vi "MasterSlaveDAQ.vi"() -> ()   [LabVIEW 2014]
doc: "Use this template to build a user interface event handler design pattern. Use this pattern for dialog boxes and other user interfaces. You also can create and execute user-defined events that the VI can handle the same way as user interface events."
uses:
  subVIs/MasterState.ctl
  subVIs/SlaveStateData.ctl
  subVIs/SlaveState.ctl
  <vilib>/Utility/error.llb/DialogType.ctl
  <vilib>/DAQmx/create/channels.llb/DAQmx Create Channel (AI-Voltage-Basic).vi
  <vilib>/DAQmx/configure/timing.llb/DAQmx Timing (Sample Clock).vi
  <vilib>/DAQmx/read.llb/DAQmx Read (Analog Wfm 1Chan NSamp).vi
  <resource>/objmgr/daqmx.rc
panel:
  in  "File Path":path
  in  "Acquire Data":bool
  in  "Log Data":bool
  in  "File Comment":string
  in  "DAQ Parameters":T1={"physical channels"="", "maximum value"=5.0, "minimum value"=-5.0, "rate"=1000.0, "read period"=0.5} {"read period" format="%0.2f"; "rate" format="%0.2f"; "minimum value" format="%0.2f"; "maximum value" format="%0.2f"}
  out "Waveform Chart":waveform(dbl)(graph)
  in  "quit":bool
  # "V"
  # "V"
  # "Hz"
  # "s"
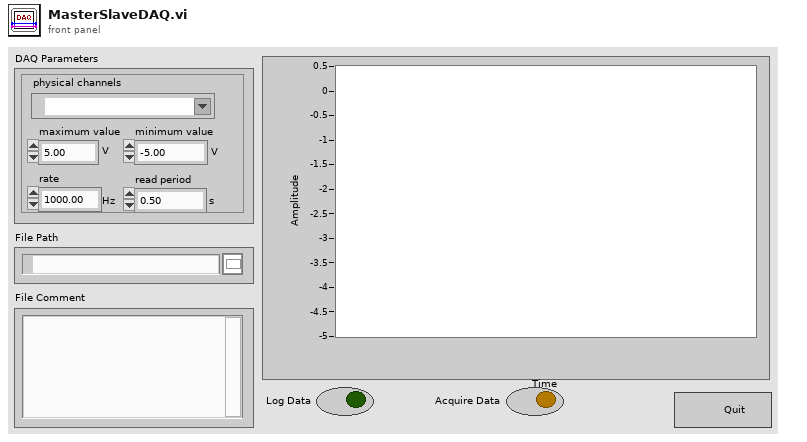
[diagram p1: front panel]
types:
  T1 = cluster{"physical channels":tag, "maximum value":dbl, "minimum value":dbl, "rate":dbl, "read period":dbl}
  T2 = typedef "SlaveState.ctl" = enum16{"Init", "Idle", "CheckError", "Finalize", "StartDAQ", "AcquireAndLog", "StopDAQ", "UpdateFile"}
  T3 = typedef "SlaveStateData.ctl" = cluster{"New State":T2, "DAQ Ref":refnum<k21>, "File Ref":refnum<file>}
  T4 = typedef "MasterState.ctl" = enum16{"Init", "Idle", "CheckError", "Finalize", "ConfigDAQ", "StartDAQ", "AcquireAndLog", "StopDAQ", "ClearDAQ", "OpenFile", "CloseFile"}
  T5 = typedef "DialogType.ctl" = u16
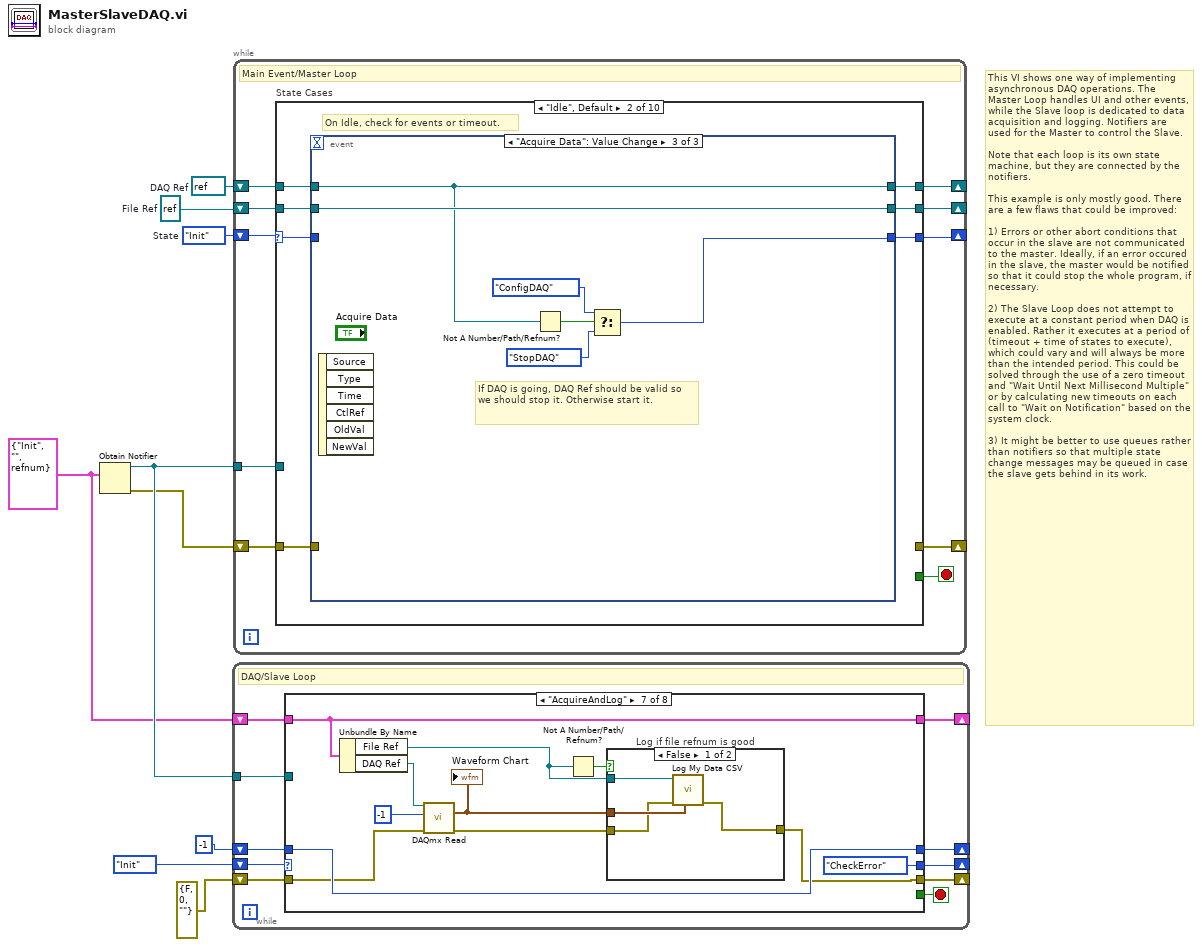
[diagram p0: block diagram]
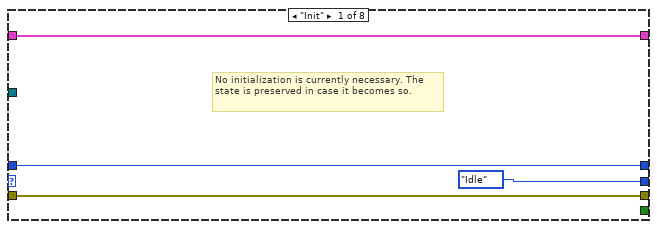
[diagram p2: hidden frame]
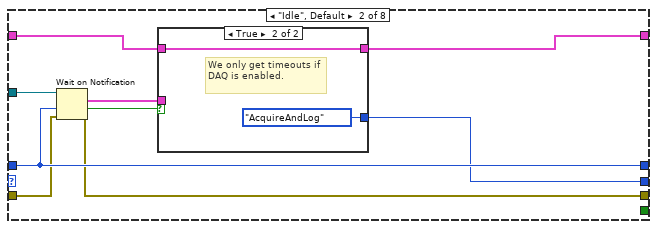
[diagram p3: hidden frame]
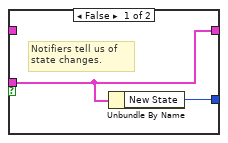
[diagram p4: hidden frame]
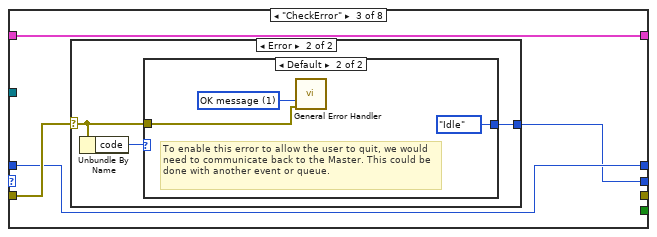
[diagram p5: hidden frame]
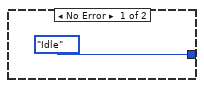
[diagram p6: hidden frame]
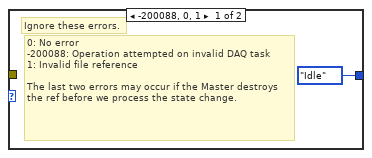
[diagram p7: hidden frame]
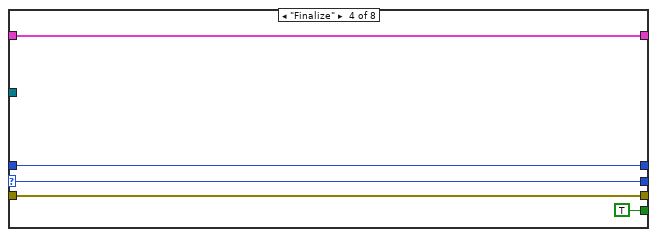
[diagram p8: hidden frame]
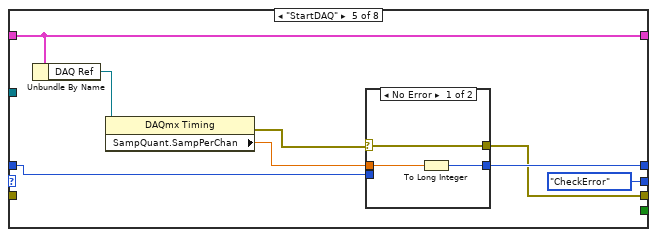
[diagram p9: hidden frame]
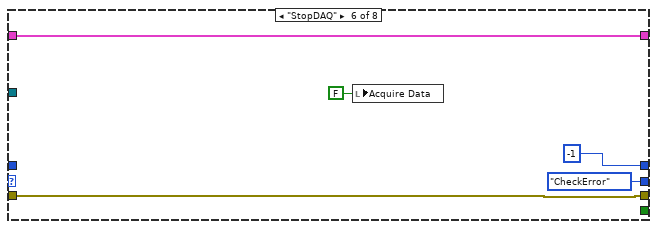
[diagram p11: hidden frame]
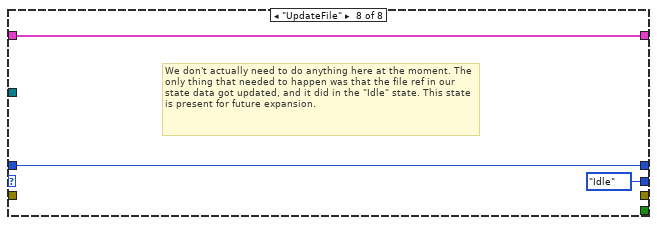
[diagram p13: hidden frame]
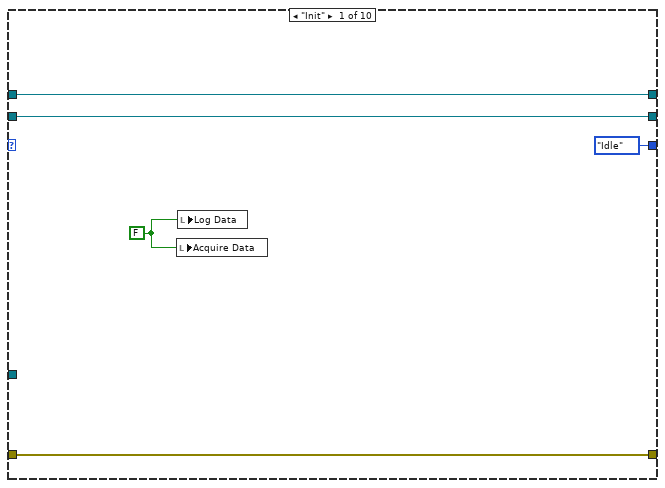
[diagram p14: hidden frame]
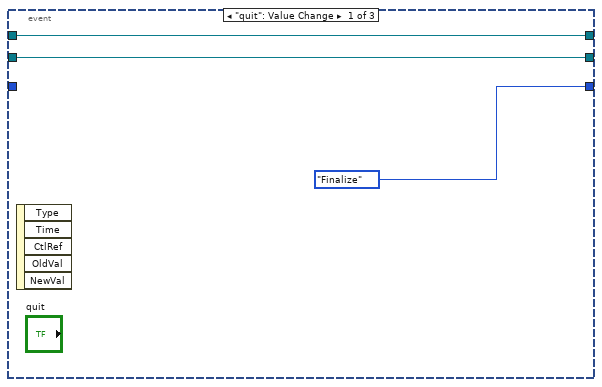
[diagram p15: hidden frame]
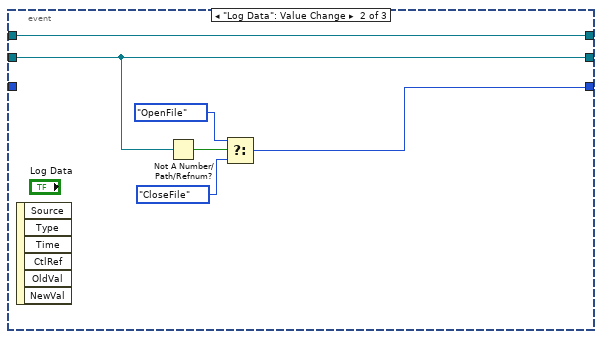
[diagram p16: hidden frame]
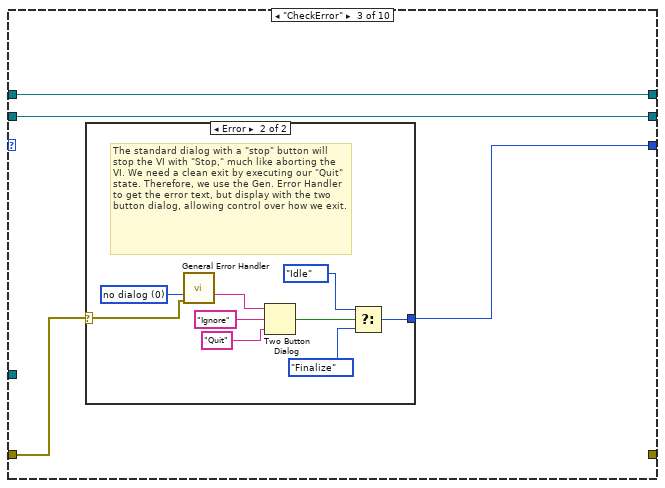
[diagram p17: hidden frame]
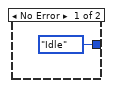
[diagram p18: hidden frame]
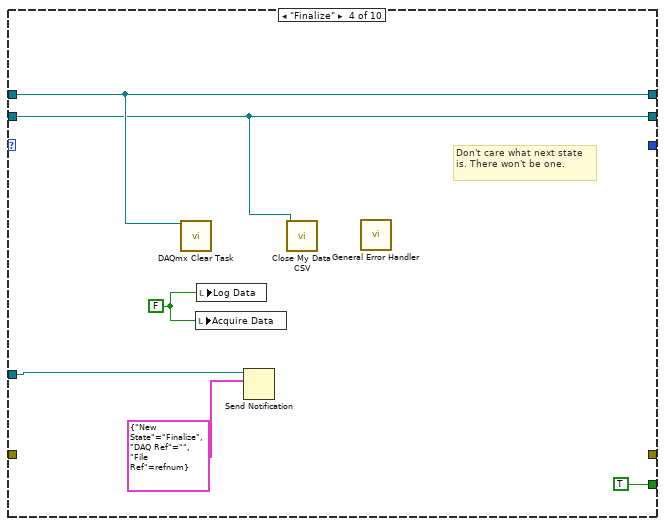
[diagram p19: hidden frame]
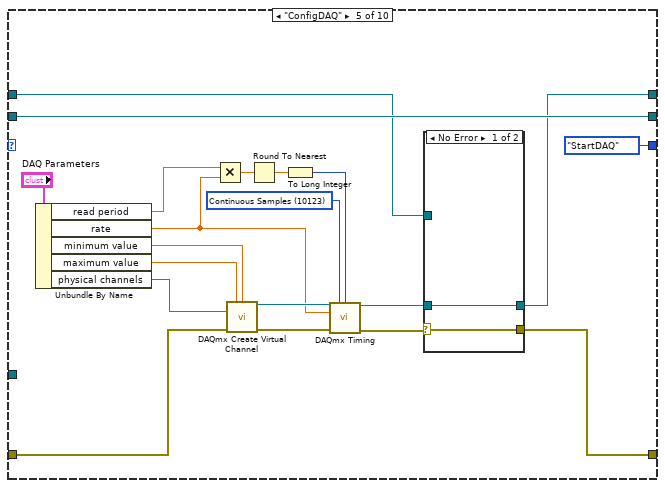
[diagram p20: hidden frame]
diagram:
  w4 = T3 {"New State"=enum."Init", "DAQ Ref"="", "File Ref"=refnum}
  w7 = refnum<file> refnum  # File Ref
  w8 = refnum<k21> refnum  # DAQ Ref
  w9 = MasterState."Init"  # State
  # "This VI shows one way of implementing asynchronous DAQ operations. The Master Loop handles UI and other events, while the Slave loop is dedicated to data acquisition and logging. Notifiers are used for the Master to control the Slave.\n\nNote that each loop is its own state machine, but they are connected by the notifiers.\n\nThis example is only mostly good. There are a few flaws that could be improved:\n\n1) Errors or other abort conditions that occur in the slave are not communicated to the master. Ideally, if an error occured in the slave, the master would be notified so that it could stop the whole program, if necessary.\n\n2) The Slave Loop does not attempt to execute at a constant period when DAQ is enabled. Rather it executes at a period of (timeout + time of states to execute), which could vary and will always be more than the intended period. This could be solved through the use of a zero timeout and \"Wait Until Next Millisecond Multiple\" or by calculating new timeouts on each call to \"Wait on Notification\" based on the system clock.\n\n3) It might be better to use queues rather than notifiers so that multiple state change messages may be queued in case the slave gets behind in its work."
  n1 = Obtain Notifier(notification data type=w4) -> (notifier out=w6:refnum<notifier>, error out=w2:errorcluster)  [unwired: 3 in, 1 out]
  n2 = while {
    tunnel: w6 -> [w18]
    shift-right: [w17] -> _
    shift-left: SlaveState."Init" ("State") -> [w19]
    shift-right: [w13] -> _
    shift-left: w4 -> [w16]
    shift-right: [w14] -> _
    shift-left: -1 -> [w15]
    shift-right: [w11] -> _
    shift-left: errorcluster {"status"=FALSE, "code"=0, "source"=""} ("error out") -> [w12]
    stop <- w10 stop-if-true
    # "DAQ/Slave Loop"
    n3 = case shown="\"AcquireAndLog\"" w19 {
      selector: w19 -> [_ _ _ w50 _ _ _ _]
      tunnel: w18 -> [_ w32 _ _ _ _ _ _]
      tunnel: [SlaveState."Idle" ("New State") w25 w37 w50 SlaveState."CheckError" ("State") SlaveState."CheckError" ("State") SlaveState."CheckError" ("State") SlaveState."Idle" ("State")] -> w17
      tunnel: w16 -> [w21 w27 w40 w52 w57 w71 w76 w90]
      tunnel: w15 -> [w22 w31 w38 w51 w59 _ w77 w89]
      tunnel: [w22 w31 w38 w51 w60 -1 w77 w89] -> w14
      tunnel: [w21 w24 w40 w52 w57 w71 w76 w90] -> w13
      tunnel: w12 -> [w20 w29 w39 w49 _ w67 w74 _]
      tunnel: [w20 w30 _ w49 w58 w67 w73 _] -> w11
      tunnel: [_ _ _ TRUE _ _ _ _] -> w10
      frame "Init" {
        # "No initialization is currently necessary. The state is preserved in case it becomes so."
      }
      frame "Idle", Default {
        n4 = Wait on Notification(notifier=w32, timeout in ms (-1)=w31, error in (no error)=w29) -> (notification=w26:T3, timed out?=w28:bool, error out=w30:errorcluster)  [unwired: 1 in, 1 out]
        n5 = case shown="True" w28 {
          tunnel: w27 -> [_ w36]
          tunnel: w26 -> [w33 _]
          tunnel: [w34 SlaveState."AcquireAndLog" ("New State")] -> w25
          tunnel: [w33 w36] -> w24
          frame False {
            # "Notifiers tell us of state changes."
            n6 = Unbundle By Name(w33) -> ("New State"=w34:T2)
          }
          frame True {
            # "We only get timeouts if DAQ is enabled."
          }
        }
      }
      frame "CheckError" {
        n7 = case shown="Error" w39 {
          selector: w39 -> [_ w43]
          tunnel: [SlaveState."Idle" ("State") w44] -> w37
          frame No Error {
          }
          frame Error {
            n8 = Unbundle By Name(w43) -> ("code"=w42:i32)
            n9 = case shown="Default" w42 {
              tunnel: [SlaveState."Idle" ("State") SlaveState."Idle" ("State")] -> w44
              tunnel: w43 -> [_ w47]
              frame -200088, 0, 1 {
                # "0: No error\n-200088: Operation attempted on invalid DAQ task\n1: Invalid file reference\n\nThe last two errors may occur if the Master destroys the ref before we process the state change."
                # "Ignore these errors."
              }
              frame Default {
                w48 = T5 1 items=["no dialog", "OK message", "continue or stop message", "OK message + warnings", "continue/stop + warnings"] ("type of dialog (OK msg:1)")
                # "To enable this error to allow the user to quit, we would need to communicate back to the Master. This could be done with another event or queue."
                n10 = call <vilib>:"General Error Handler.vi"("type of dialog (OK msg:1)"=w48, "error in (no error)"=w47) -> ()  [unwired: 9 in, 5 out]
              }
            }
          }
        }
      }
      frame "Finalize" {
      }
      frame "StartDAQ" {
        n11 = Unbundle By Name(w57) -> ("DAQ Ref"=w56:refnum<k21>)
        n12 = property class="DAQmx Timing"(reference=w56) -> (error out=w54:errorcluster, "SampQuant.SampPerChan"=w61:dbl)  [unwired: 1 in, 1 out]
        n13 = case shown="No Error" w54 {
          selector: w54 -> [w62 w66]
          tunnel: w61 -> [w64 _]
          tunnel: [w63 w65] -> w60
          tunnel: [w62 w66] -> w58
          tunnel: w59 -> [_ w65]
          frame No Error {
            n14 = To Long Integer(number=w64) -> (32bit integer=w63:i32)
          }
          frame Error {
          }
        }
      }
      frame "StopDAQ" {
        n15 = local write "Acquire Data"(FALSE ("Acquire Data")) -> ()
      }
      frame "AcquireAndLog" {
        n16 = Unbundle By Name(w76) -> ("File Ref"=w72:refnum<file>, "DAQ Ref"=w75:refnum<k21>)
        n17 = call-poly <vilib>:"DAQmx Read.vi"("task/channels in"=w75, "number of samples per channel"=-1, "error in"=w74) -> ("data"=w78:waveform(dbl), "error out"=w79:errorcluster)  [unwired: 10 in, 1 out]
        "Waveform Chart" <- w78
        n18 = Not A Number/Path/Refnum?(number/path/refnum=w72) -> (NaN/Path/Refnum?=w80:bool)
        n19 = case "Log if file refnum is good" shown="False" w80 {
          tunnel: w79 -> [w83 w87]
          tunnel: w72 -> [w86 _]
          tunnel: w78 -> [w85 _]
          tunnel: [w84 w87] -> w73
          frame False {
            n20 = call "Log My Data CSV.vi"("Data"=w85, "error in"=w83, "file refnum"=w86) -> ("error out"=w84:errorcluster)  [unwired: 7 in, 1 out]
          }
          frame True {
          }
        }
      }
      frame "UpdateFile" {
        # "We don't actually need to do anything here at the moment. The only thing that needed to happen was that the file ref in our state data got updated, and it did in the \"Idle\" state. This state is present for future expansion."
      }
    }
  }
  n21 = while {
    shift-right: [w99] -> _
    shift-left: w9 -> [w100]
    shift-right: [w98] -> _
    shift-left: w8 -> [w97]
    shift-right: [w96] -> _
    shift-left: w7 -> [w95]
    shift-right: [w94] -> _
    shift-left: w2 -> [w93]
    tunnel: w6 -> [w91]
    stop <- w92 stop-if-true
    # "Main Event/Master Loop"
    n22 = case "State Cases" shown="\"Idle\", Default" w100 {
      selector: w100 -> [_ w112 _ _ _ _ _ _ _ _]
      tunnel: [MasterState."Idle" ("State") w111 w129 _ MasterState."StartDAQ" ("State") MasterState."CheckError" ("State") MasterState."ClearDAQ" ("State") MasterState."CheckError" ("State") MasterState."CheckError" ("State") MasterState."CheckError" ("State")] -> w99
      tunnel: [w105 w108 w131 w146 w158 w174 w188 refnum<k21> refnum ("DAQ Ref") w204 w230] -> w98
      tunnel: w97 -> [w105 w107 w131 w146 w159 w174 w188 w198 w204 w230]
      tunnel: [w104 w110 w130 w145 w167 w177 w195 w200 w215 w234] -> w96
      tunnel: w95 -> [w104 w109 w130 w145 w167 w177 w195 w200 w205 w237]
      tunnel: [w101 _ _ _ w156 w178 w190 w196 w214 w227] -> w94
      tunnel: w93 -> [w101 w106 w128 _ w148 w175 w187 w197 w211 w233]
      tunnel: [_ _ _ TRUE _ _ _ _ _ _] -> w92
      tunnel: w91 -> [_ _ _ w143 _ w182 w194 _ w208 w226]
      frame "Init" {
        w102 = FALSE
        n23 = local write "Acquire Data"(w102) -> ()
        n24 = local write "Log Data"(w102) -> ()
      }
      frame "Idle", Default {
        # "On Idle, check for events or timeout."
        # "States"
        n25 = event shown="[2] \"Acquire Data\": Value Change" {
          selector: _ -> [_ _ _]
          dyn-events: _ -> [_ _ _]
          timeout: _ -> [_ _ _]
          tunnel: w112 -> [_ _ _]
          tunnel: [MasterState."Finalize" ("State") w116 w122] -> w111
          tunnel: [w114 w119 w127] -> w110
          tunnel: w109 -> [w114 w119 w127]
          tunnel: [w115 w121 w125] -> w108
          tunnel: w107 -> [w115 w121 w125]
          tunnel: w106 -> [_ _ _]
          event "quit": Value Change {
            n26 = event-data() -> ()  [unwired: 1 in, 5 out]
          }
          event "Log Data": Value Change {
            n27 = event-data() -> ()  [unwired: 1 in, 6 out]
            n28 = Not A Number/Path/Refnum?(number/path/refnum=w119) -> (NaN/Path/Refnum?=w120:bool)
            n29 = Select(t=MasterState."OpenFile" ("State"), s=w120, f=MasterState."CloseFile" ("State")) -> (s? t:f=w116:T4)
          }
          event "Acquire Data": Value Change {
            # "If DAQ is going, DAQ Ref should be valid so we should stop it. Otherwise start it."
            n30 = event-data() -> ()  [unwired: 1 in, 6 out]
            n31 = Not A Number/Path/Refnum?(number/path/refnum=w125) -> (NaN/Path/Refnum?=w126:bool)
            n32 = Select(t=MasterState."ConfigDAQ" ("State"), s=w126, f=MasterState."StopDAQ" ("State")) -> (s? t:f=w122:T4)
          }
        }
      }
      frame "CheckError" {
        n33 = case shown="Error" w128 {
          selector: w128 -> [_ w133]
          tunnel: [MasterState."Idle" ("State") w134] -> w129
          frame No Error {
          }
          frame Error {
            w141 = T5 0 items=["no dialog", "OK message", "continue or stop message", "OK message + warnings", "continue/stop + warnings"] ("type of dialog (OK msg:1)")
            # "The standard dialog with a \"stop\" button will stop the VI with \"Stop,\" much like aborting the VI. We need a clean exit by executing our \"Quit\" state. Therefore, we use the Gen. Error Handler to get the error text, but display with the two button dialog, allowing control over how we exit."
            n34 = call <vilib>:"General Error Handler.vi"("type of dialog (OK msg:1)"=w141, "error in (no error)"=w133) -> ("message"=w140:string)  [unwired: 9 in, 4 out]
            n35 = Two Button Dialog(message=w140, 1:"Quit" ("F button name (\"Cancel\")"), 2:"Ignore" ("T button name (\"OK\")")) -> (T button?=w137:bool)
            n36 = Select(t=MasterState."Idle" ("State"), s=w137, f=MasterState."Finalize" ("State")) -> (s? t:f=w134:T4)
          }
        }
      }
      frame "Finalize" {
        w144 = FALSE
        # "Don't care what next state is. There won't be one."
        n37 = call <vilib>:"DAQmx Clear Task.vi"("task in"=w146) -> ()  [unwired: 14 in, 1 out]
        n38 = local write "Acquire Data"(w144) -> ()
        n39 = local write "Log Data"(w144) -> ()
        n40 = Send Notification(notification=T3 {"New State"=enum."Finalize", "DAQ Ref"="", "File Ref"=refnum}, notifier=w143) -> ()  [unwired: 1 in, 2 out]
        n41 = call "Close My Data CSV.vi"("file refnum"=w145) -> ()  [unwired: 10 in, 1 out]
        n42 = call <vilib>:"General Error Handler.vi"() -> ()  [unwired: 11 in, 5 out]
      }
      frame "ConfigDAQ" {
        w164 = 10123 items=["Finite Samples"=10178, "Continuous Samples"=10123, "Hardware Timed Single Point"=12522] ("sample mode")
        n43 = Unbundle By Name("DAQ Parameters") -> ("read period"=w153:dbl, "rate"=w152:dbl, "minimum value"=w151:dbl, "maximum value"=w150:dbl, "physical channels"=w149:tag)
        n44 = Multiply(x=w153, y=w152) -> (x*y=w163:dbl)
        n45 = call-poly <vilib>:"DAQmx Create Virtual Channel.vi"("maximum value"=w150, "minimum value"=w151, "physical channels"=w149, "error in"=w148) -> ("task out"=w166:refnum<k21>, "error out"=w165:errorcluster)  [unwired: 10 in]
        n46 = Round To Nearest(number=w163) -> (nearest integer value=w162:dbl)
        n47 = To Long Integer(number=w162) -> (32bit integer=w161:i32)
        n48 = call-poly <vilib>:"DAQmx Timing.vi"("task/channels in"=w166, "sample mode"=w164, "samples per channel"=w161, "rate"=w152, "error in"=w165) -> ("task out"=w157:refnum<k21>, "error out"=w160:errorcluster)  [unwired: 9 in]
        n49 = case shown="No Error" w160 {
          selector: w160 -> [w168 w171]
          tunnel: w159 -> [_ w170]
          tunnel: [w169 w170] -> w158
          tunnel: w157 -> [w169 _]
          tunnel: [w168 w171] -> w156
          frame No Error {
          }
          frame Error {
          }
        }
      }
      frame "StartDAQ" {
        # "Set \"StartDAQ\" State on slave"
        n50 = call <vilib>:"DAQmx Start Task.vi"("task/channels in"=w174, "error in"=w175) -> ("error out"=w173:errorcluster)  [unwired: 12 in, 1 out]
        n51 = Bundle By Name(cluster=T3 {"New State"=enum."Init", "DAQ Ref"="", "File Ref"=refnum} ("notification"), "File Ref"=w177, "New State"=SlaveState."StartDAQ", "DAQ Ref"=w174) -> (w179:T3)
        n52 = Send Notification(notification=w179, notifier=w182, error in (no error)=w173) -> (error out=w178:errorcluster)  [unwired: 1 out]
        n53 = case shown="No Error" w173 {
          tunnel: [TRUE FALSE] -> w172
          frame No Error {
          }
          frame Error {
          }
        }
        n54 = local write "Acquire Data"(w172) -> ()
      }
      frame "StopDAQ" {
        n55 = call <vilib>:"DAQmx Stop Task.vi"("task/channels in"=w188, "error in"=w187) -> ("error out"=w186:errorcluster)  [unwired: 12 in, 1 out]
        n56 = Bundle By Name(cluster=T3 {"New State"=enum."Init", "DAQ Ref"="", "File Ref"=refnum} ("notification"), "New State"=SlaveState."StopDAQ", "DAQ Ref"=refnum<k21> refnum) -> (w191:T3)
        n57 = Send Notification(notification=w191, notifier=w194, error in (no error)=w186) -> (error out=w190:errorcluster)  [unwired: 1 out]
      }
      frame "ClearDAQ" {
        n58 = call <vilib>:"DAQmx Clear Task.vi"("task in"=w198, "error in"=w197) -> ("error out"=w196:errorcluster)  [unwired: 13 in]
      }
      frame "OpenFile" {
        # "Open new log file"
        # "Inform slave of new log file"
        n59 = Get Date/Time In Seconds() -> (seconds since 1Jan1904=w218:timestamp)
        n60 = call "Open My Data CSV.vi"("Comment"="File Comment", "Time Stamp"=w218, "error in"=w211, "file path"="File Path") -> ("error out"=w210:errorcluster, "refnum out"=w203:refnum<file>)  [unwired: 6 in]
        n61 = Bundle By Name(cluster=T3 {"New State"=enum."Init", "DAQ Ref"="", "File Ref"=refnum} ("notification"), "New State"=SlaveState."UpdateFile", "DAQ Ref"=w204, "File Ref"=w203) -> (w202:T3)
        n62 = Send Notification(notification=w202, notifier=w208, error in (no error)=w210) -> (error out=w209:errorcluster)  [unwired: 1 out]
        n63 = case shown="No Error" w209 {
          selector: w209 -> [w220 w224]
          tunnel: [w221 w222] -> w215
          tunnel: w203 -> [w221 _]
          tunnel: [w220 w224] -> w214
          tunnel: [TRUE ("Log Data") FALSE ("Log Data")] -> w213
          tunnel: w205 -> [_ w222]
          frame No Error {
          }
          frame Error {
          }
        }
        n64 = local write "Log Data"(w213) -> ()
      }
      frame "CloseFile" {
        w229 = refnum<file> refnum  # File Ref
        w234 = refnum<file> refnum  # File Ref
        # "Close file"
        # "Inform slave of closed file"
        n65 = call "Close My Data CSV.vi"("error in"=w233, "file refnum"=w237) -> ("error out"=w228:errorcluster)  [unwired: 9 in]
        n66 = Bundle By Name(cluster=T3 {"New State"=enum."Init", "DAQ Ref"="", "File Ref"=refnum} ("notification"), "New State"=SlaveState."UpdateFile", "DAQ Ref"=w230, "File Ref"=w229) -> (w225:T3)
        n67 = Send Notification(notification=w225, notifier=w226, error in (no error)=w228) -> (error out=w227:errorcluster)  [unwired: 1 out]
        n68 = local write "Log Data"(FALSE ("Log Data")) -> ()
      }
    }
  }
